vi "Author Data Extractor.vi"(8 "Error In":errorcluster, 10 "Author Data":variant[][](array[variant])=[[variant]], 11 "Author Initials":string) -> (0 "Error Out":errorcluster, 2 "Exists?":bool, 3 "Author Information":T1)   [LabVIEW 2020]
uses:
  <vilib>/addons/database/_DB Variant To Data/Database Variant To Data.xnode
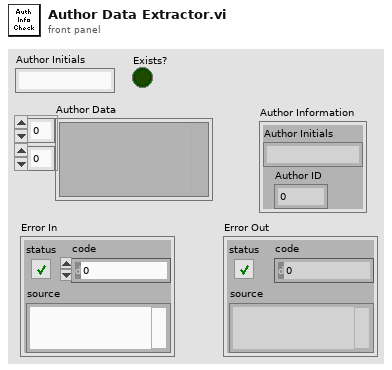
[diagram p1: front panel]
types:
  T1 = cluster{"Author Initials":string, "Author ID":i32}
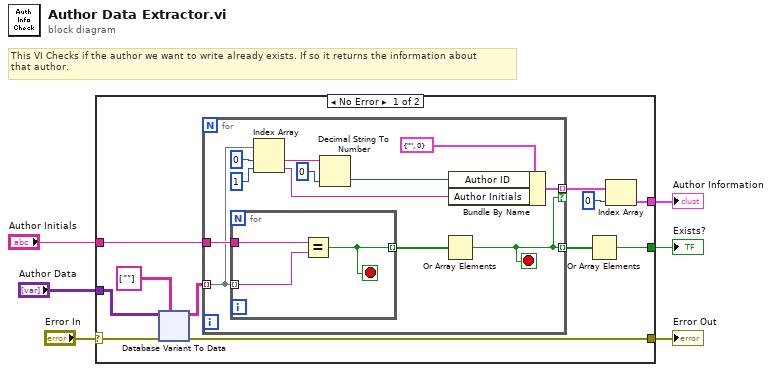
[diagram p0: block diagram]
diagram:
  # "This VI Checks if the author we want to write already exists. If so it returns the information about\nthat author."
  n1 = case shown="No Error" "Error In" {
    selector: "Error In" -> [w13 w77]
    tunnel: "Author Data" -> [w14 _]
    tunnel: "Author Initials" -> [w12 _]
    tunnel: [w10 _] -> w3
    tunnel: [w7 _] -> w1
    tunnel: [w11 w77] -> w2
    frame No Error {
      n2 = xnode "Database Variant To Data"("database variant"=w14, "error in (no error)"=w13, "type"=string[][] [[""]] ("columns")) -> ("data"=w15:string[][], "error out"=w11:errorcluster)
      n3 = for {
        tunnel: w15 -> [w27] mode=indexing
        tunnel: w12 -> [w29]
        tunnel: [w18] -> w16 mode=indexing
        tunnel: [w19] -> w9 mode=indexing if=w18
        stop <- w18 stop-if-true
        n4 = for {
          tunnel: w27 -> [w31] mode=indexing
          tunnel: w29 -> [w32]
          tunnel: [w30] -> w28 mode=indexing
          stop <- w30 stop-if-true
          n5 = Equal?(x=w32, y=w31) -> (x = y?=w30:bool)
        }
        n6 = Index Array(array=w27, index #1=0 ("index"), index #2=1 ("index")) -> (element #1=w24:string, element #2=w21:string)
        n7 = Decimal String To Number(string=w24, default (0L)=0 ("default (0 I32)")) -> (number=w20:i32)  [unwired: 1 in, 1 out]
        n8 = Or Array Elements(Boolean array=w28) -> (logical OR=w18:bool)
        n9 = Bundle By Name(cluster=T1 {"Author Initials"="", "Author ID"=0} ("output cluster"), "Author ID"=w20, "Author Initials"=w21) -> (w19:T1)
      }
      n10 = Or Array Elements(Boolean array=w16) -> (logical OR=w10:bool)
      n11 = Index Array(array=w9, index=0) -> (element=w7:T1)
    }
    frame Error {
    }
  }
  "Exists?" <- w3
  "Error Out" <- w2
  "Author Information" <- w1
